vi "Create Stack Info.vi"(7 "nFrames":u32, 8 "error in (no error)":errorcluster, 9 "Camera Settings":T2={"Exposure Time (ms)"=100.0, "Binning"=enum."2x2", "Scan Mode"=0, "Frames to Acquire"=1000.0, "Pixel Correction"=FALSE, "Frames to Skip"=0, "File Path"=path "", "Duty cycle"=0.0, "ALEX"=FALSE, "Shutter Enable"=[], "Timelapse Interval (s)"=0} {"Timelapse Interval (s)" max=60000 step=1; "Exposure Time (ms)" min=1.0 max=10000.0 step=1.0}, 11 "Virtual Camera in":refnum<class "Virtual Camera.lvclass">) -> (0 "error out":errorcluster, 2 "Stack Info":T1, 3 "Virtual Camera out":refnum<class "Virtual Camera.lvclass">)   [LabVIEW 2018, in "Virtual Camera.lvlib" / "Virtual Camera.lvclass"]
uses:
  Virtual Camera.lvclass
  Resources/Type Defs/Camera Settings.ctl
  Resources/GLOBAL/GLOBAL Experiment Metadata.vi
  Resources/GLOBAL/GLOBAL Time-critical.vi
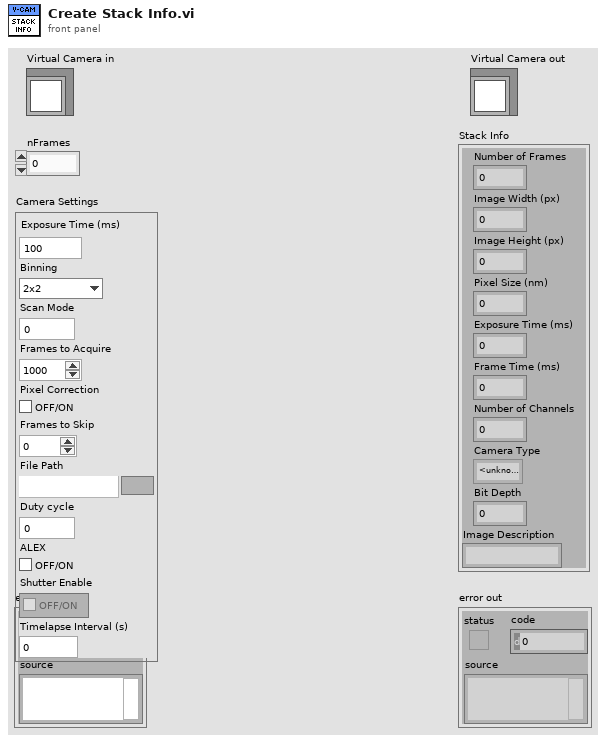
[diagram p1: front panel]
types:
  T1 = cluster{"Number of Frames":u32, "Image Width (px)":u32, "Image Height (px)":u32, "Pixel Size (nm)":dbl, "Exposure Time (ms)":dbl, "Frame Time (ms)":dbl, "Number of Channels":u32, "Camera Type":enum16{"<unknown>", "Evolve 512", "Orca-Flash 4.0 V2"}, "Bit Depth":u32, "Image Description":string}
  T2 = typedef "Camera Settings.ctl" = cluster{"Exposure Time (ms)":dbl, "Binning":enum16{"1x1", "2x2", "4x4"}, "Scan Mode":i32, "Frames to Acquire":dbl, "Pixel Correction":bool, "Frames to Skip":u32, "File Path":path, "Duty cycle":dbl, "ALEX":bool, "Shutter Enable":bool[], "Timelapse Interval (s)":u32}
  T3 = enum16{"<unknown>", "Evolve 512", "Orca-Flash 4.0 V2"}
  T4 = cluster{"Shutter Enable":bool[], "Duty Cycle":dbl, "Wavelengths":dbl[], "ALEX?":bool}
  T5 = typedef "Physical Camera Assignment.ctl" = cluster{"Channel Name":string, "Camera Type":T6, "Serial Number":string, "Flip Vertically":bool, "Flip Horizontally":bool, "photonsPerCount":dbl, "wavelength":i16}
  T6 = typedef "Camera Type.ctl" = enum16{"Hamamatsu"}
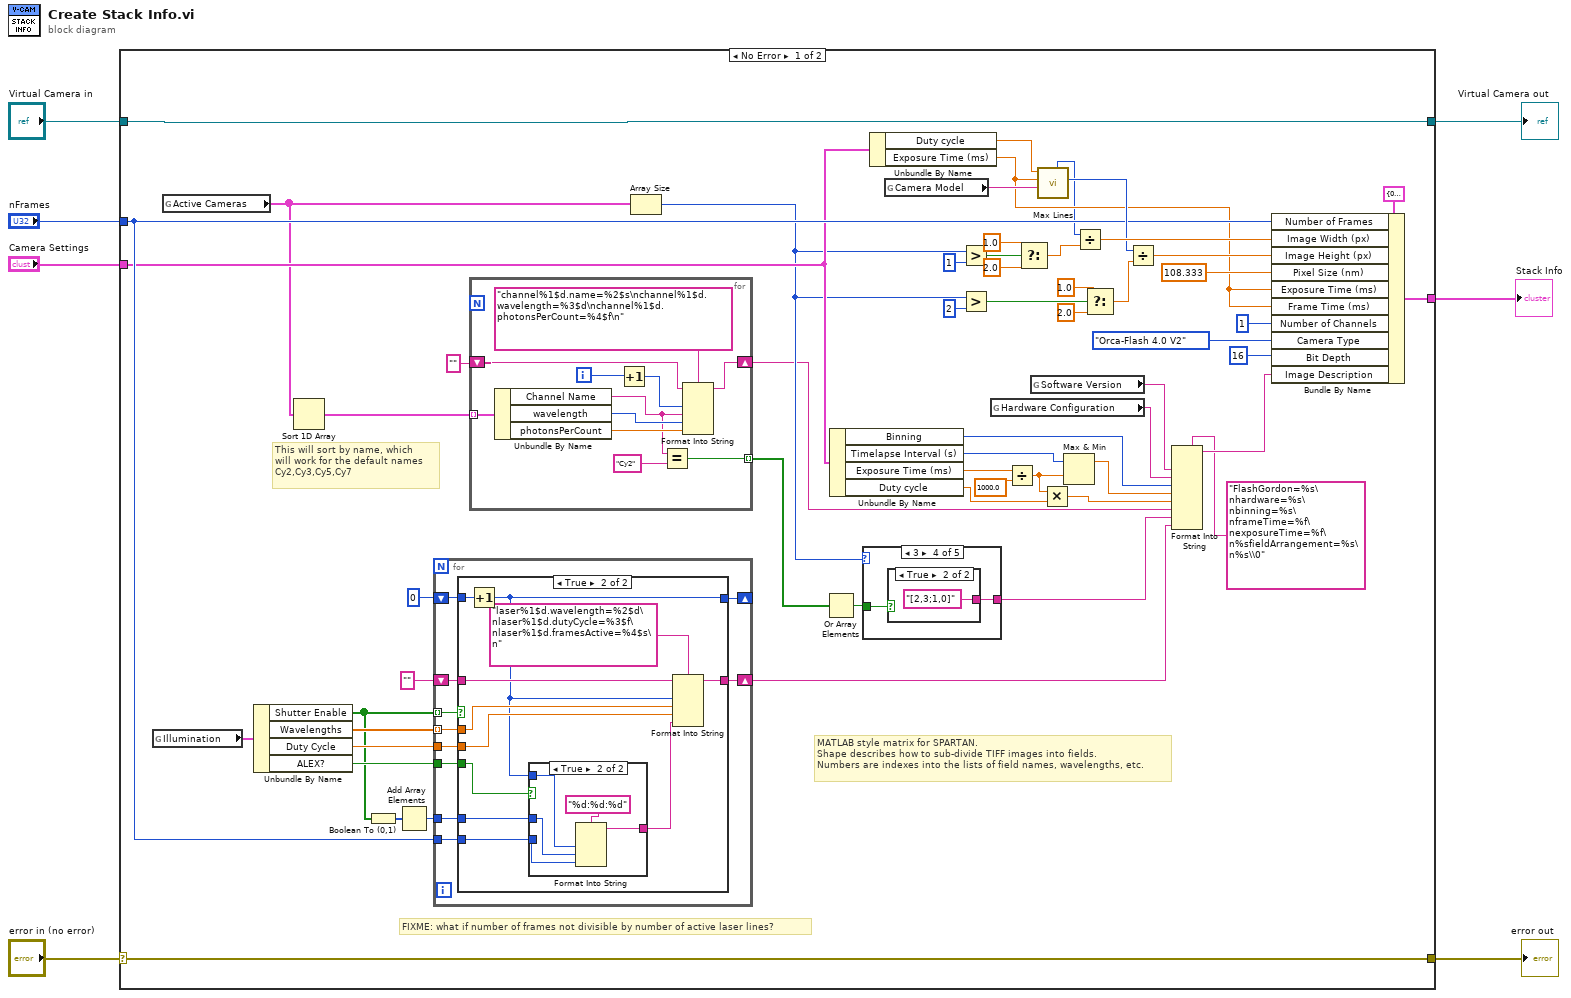
[diagram p0: block diagram]
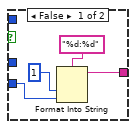
[diagram p3: hidden frame]
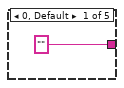
[diagram p4: hidden frame]
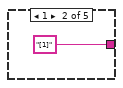
[diagram p5: hidden frame]
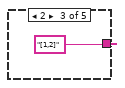
[diagram p6: hidden frame]
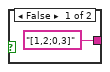
[diagram p7: hidden frame]
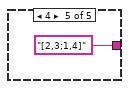
[diagram p8: hidden frame]
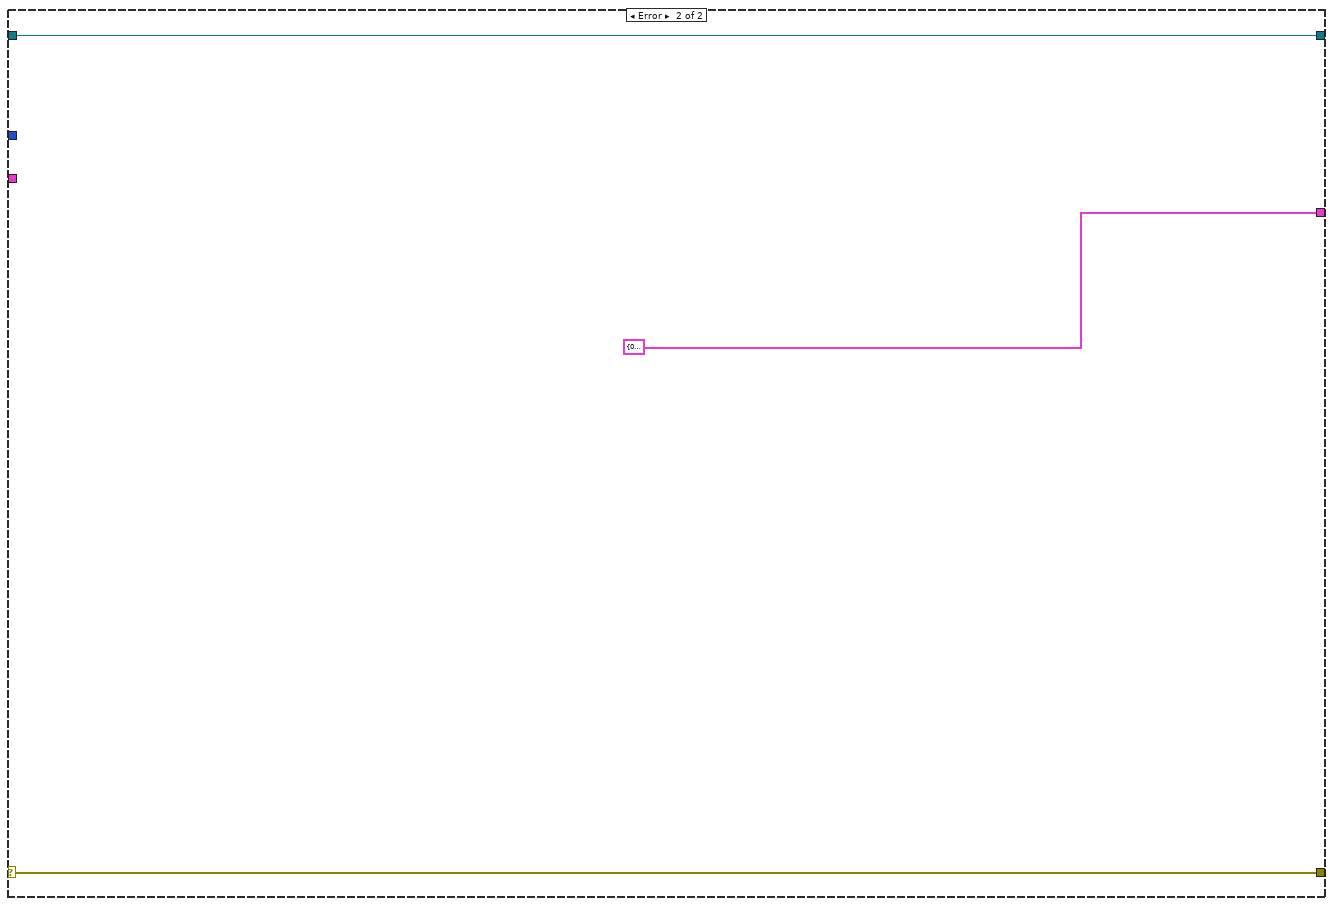
[diagram p9: hidden frame]
diagram:
  n1 = case shown="No Error" "error in (no error)" {
    selector: "error in (no error)" -> [w64 w118]
    tunnel: [w64 w118] -> w6
    tunnel: [w43 w117] -> w4
    tunnel: "Virtual Camera in" -> [w43 w117]
    tunnel: "Camera Settings" -> [w21 _]
    tunnel: "nFrames" -> [w25 _]
    tunnel: [w44 T1 {"Number of Frames"=0, "Image Width (px)"=0, "Image Height (px)"=0, "Pixel Size (nm)"=0.0, "Exposure Time (ms)"=0.0, "Frame Time (ms)"=0.0, "Number of Channels"=0, "Camera Type"=enum."<unknown>", "Bit Depth"=0, "Image Description"=""} ("Stack Info")] -> w1
    frame No Error {
      # "FIXME: what if number of frames not divisible by number of active laser lines?"
      # "MATLAB style matrix for SPARTAN.\nShape describes how to sub-divide TIFF images into fields.\nNumbers are indexes into the lists of field names, wavelengths, etc."
      # "This will sort by name, which\nwill work for the default names\nCy2,Cy3,Cy5,Cy7"
      n2 = global read "GLOBAL Experiment Metadata.vi" "Illumination"() -> (w34:T4)
      n3 = global read "GLOBAL Time-critical.vi" "Active Cameras"() -> (w20:T5[])
      n4 = Unbundle By Name(w34) -> ("Shutter Enable"=w24:bool[], "Wavelengths"=w32:dbl[], "Duty Cycle"=w33:dbl, "ALEX?"=w31:bool)
      n5 = Sort 1D Array(array=w20) -> (sorted array=w39:T5[])
      n6 = Boolean To (0,1)(Boolean=w24) -> (0, 1=w23:i16[])
      n7 = Add Array Elements(numeric array=w23) -> (sum=w22:i16)
      n8 = for {
        tunnel: w24 -> [w74] mode=indexing
        tunnel: w33 -> [w70]
        tunnel: w32 -> [w71] mode=indexing
        tunnel: w31 -> [w69]
        shift-right: [w72] -> w29
        shift-left: "" -> [w73]
        shift-right: [w67] -> _
        shift-left: 0 -> [w68]
        tunnel: w25 -> [w66]
        tunnel: w22 -> [w65]
        n9 = case shown="True" w74 {
          tunnel: w73 -> [w76 w85]
          tunnel: [w76 w86] -> w72
          tunnel: w71 -> [_ w84]
          tunnel: w70 -> [_ w83]
          tunnel: w69 -> [_ w81]
          tunnel: [w75 w80] -> w67
          tunnel: w68 -> [w75 w82]
          tunnel: w66 -> [_ w79]
          tunnel: w65 -> [_ w77]
          frame False {
            # "ignore inactive laser line"
          }
          frame True {
            n10 = Increment(x=w82) -> (x+1=w80:i32)
            n11 = case shown="True" w81 {
              tunnel: w80 -> [_ w92]
              tunnel: w79 -> [w89 w94]
              tunnel: [w90 w96] -> w78
              tunnel: w77 -> [_ w93]
              frame False {
                n12 = Format Into String(format string="%d:%d", 1 ("input 1"), w89) -> (resulting string=w90:string)  [unwired: 2 in, 1 out]
              }
              frame True {
                n13 = Format Into String(format string="%d:%d:%d", w92, w93, w94) -> (resulting string=w96:string)  [unwired: 2 in, 1 out]
              }
            }
            n14 = Format Into String(format string="laser%1$d.wavelength=%2$d\nlaser%1$d.dutyCycle=%3$f\nlaser%1$d.framesActive=%4$s\n", initial string=w85, w80, w84, w83, w78) -> (resulting string=w86:string)  [unwired: 1 in, 1 out]
          }
        }
      }
      n15 = for {
        tunnel: w39 -> [w115] mode=indexing
        shift-right: [w111] -> w15
        shift-left: "" -> [w110]
        tunnel: [w107] -> w40 mode=indexing
        i -> [w106]
        # "Write spectral channel information (for now one channel per camera)"
        n16 = Unbundle By Name(w115) -> ("Channel Name"=w108:string, "wavelength"=w114:i16, "photonsPerCount"=w113:dbl)
        n17 = Increment(x=w106) -> (x+1=w105:i32)
        n18 = Equal?(x=w108, y="Cy2" ("x")) -> (x = y?=w107:bool)
        n19 = Format Into String(format string="channel%1$d.name=%2$s\nchannel%1$d.wavelength=%3$d\nchannel%1$d.photonsPerCount=%4$f\n", initial string=w110, w105, w108, w114, w113) -> (resulting string=w111:string)  [unwired: 1 in, 1 out]
      }
      n20 = Array Size(array=w20) -> (size(s)=w19:i32)
      n21 = Or Array Elements(Boolean array=w40) -> (logical OR=w41:bool)
      n22 = Unbundle By Name(w21) -> ("Binning"=w27:enum16{"1x1", "2x2", "4x4"}, "Timelapse Interval (s)"=w11:u32, "Exposure Time (ms)"=w12:dbl, "Duty cycle"=w14:dbl)
      n23 = case shown="3" w19 {
        tunnel: w41 -> [_ _ _ w101 _]
        tunnel: ["" "[1]" "[1,2]" w100 "[2,3;1,4]"] -> w35
        frame 0, Default {
        }
        frame 1 {
        }
        frame 2 {
        }
        frame 3 {
          n24 = case shown="True" w101 {
            tunnel: ["[1,2;0,3]" "[2,3;1,0]"] -> w100
            frame False {
            }
            frame True {
            }
          }
        }
        frame 4 {
        }
      }
      n25 = Unbundle By Name(w21) -> ("Duty cycle"=w17:dbl, "Exposure Time (ms)"=w16:dbl)
      n26 = global read "GLOBAL Time-critical.vi" "Camera Model"() -> (w18:string)
      n27 = Greater?(x=w19, y=1) -> (0:w62:bool)
      n28 = Greater?(x=w19, y=2) -> (0:w60:bool)
      n29 = global read "GLOBAL Experiment Metadata.vi" "Hardware Configuration"() -> (w26:string)
      n30 = Divide(x=w12, y=1000.0) -> (x/y=w10:dbl)
      n31 = Select(t=1.0, s=w62, f=2.0) -> (s? t:f=w61:dbl)
      n32 = global read "GLOBAL Experiment Metadata.vi" "Software Version"() -> (w36:string)
      n33 = call "Max Lines.vi"("Camera Model"=w18, "Frame Time (ms)"=w16, "Duty cycle (fraction)"=w17) -> ("Max Lines"=w42:i32, "unbinned image width"=w8:i32)  [unwired: 3 in, 4 out]
      n34 = Multiply(x=w10, y=w14) -> (x*y=w13:dbl)
      n35 = Max & Min(x=w11, y=w10) -> (max(x,y)=w9:dbl)  [unwired: 1 out]
      n36 = Divide(x=w8, y=w61) -> (x/y=w63:dbl)
      n37 = Select(t=1.0, s=w60, f=2.0) -> (s? t:f=w59:dbl)
      n38 = Divide(x=w42, y=w59) -> (x/y=w58:dbl)
      n39 = Format Into String(format string="FlashGordon=%s\nhardware=%s\nbinning=%s\nframeTime=%f\nexposureTime=%f\n%sfieldArrangement=%s\n%s\\0" ("Image Description"), w36, w26, w27, w9, w13, w15, w35, w29) -> (resulting string=w46:string)  [unwired: 2 in, 1 out]
      n40 = Bundle By Name(cluster=T1 {"Number of Frames"=0, "Image Width (px)"=0, "Image Height (px)"=0, "Pixel Size (nm)"=0.0, "Exposure Time (ms)"=0.0, "Frame Time (ms)"=0.0, "Number of Channels"=0, "Camera Type"=enum."<unknown>", "Bit Depth"=0, "Image Description"=""} ("Stack Info"), "Number of Frames"=w25, "Image Width (px)"=w63, "Image Height (px)"=w58, "Pixel Size (nm)"=108.333, "Exposure Time (ms)"=w16, "Frame Time (ms)"=w16, "Number of Channels"=u32 1, "Camera Type"=T3."Orca-Flash 4.0 V2", "Bit Depth"=u32 16, "Image Description"=w46) -> (w44:T1)
    }
    frame Error {
    }
  }
  "error out" <- w6
  "Virtual Camera out" <- w4
  "Stack Info" <- w1
